vi "oa_Convert Waveform Reference Data Sample Rate (1 Channel).vi"(0 "resampled signal":cluster{"r0":dbl, "dr":dbl, "Y":dbl[]}={"r0"=0.0, "dr"=1.0, "Y"=[]} {"r0" format="%.2p"; "dr" format="%.2p"; "Y" format="%.2f"}, 5 "baseline in":cluster{"r0":dbl, "dr":dbl, "Y":dbl[]}={"r0"=0.0, "dr"=1.0, "Y"=[]} {"r0" format="%.2p"; "dr" format="%.2p"; "Y" format="%.2f"}, 11 "error out in":errorcluster) -> (4 "resampled signal dup":cluster{"r0":dbl, "dr":dbl, "Y":dbl[]}={"r0"=0.0, "dr"=1.0, "Y"=[]} {"r0" format="%.2p"; "dr" format="%.2p"; "Y" format="%.2f"}, 6 "baseline in out":cluster{"r0":dbl, "dr":dbl, "Y":dbl[]}={"r0"=0.0, "dr"=1.0, "Y"=[]} {"r0" format="%.2p"; "dr" format="%.2p"; "Y" format="%.2f"}, 15 "error out":errorcluster)   [LabVIEW 2017, in "SoundVib_RefDataProcess.lvlib"]
uses:
  <vilib>/addons/Sound and Vibration/Order Analysis/Referece Data Processing/SoundVib_RefDataProcess.lvlib
  <vilib>/measure/maresamp.llb/Resample Waveform (single shot).vi
  <vilib>/measure/NI_MAPro.lvlib
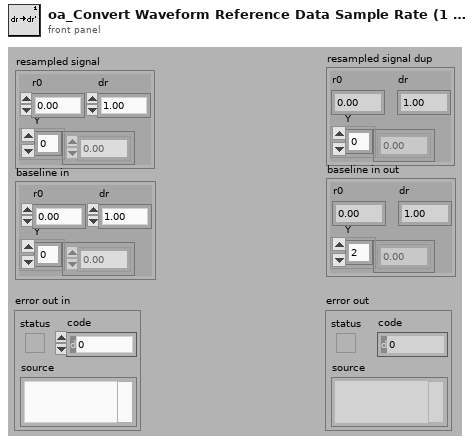
[diagram p1: front panel]
types:
  T1 = cluster{"alias rejection (dB)":dbl, "normalized bandwidth":dbl}
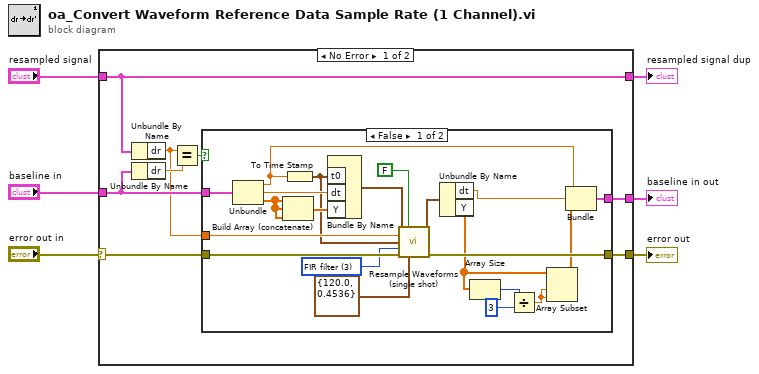
[diagram p0: block diagram]
diagram:
  n1 = case shown="No Error" "error out in" {
    selector: "error out in" -> [w12 w40]
    tunnel: [w11 w40] -> w5
    tunnel: "resampled signal" -> [w14 w39]
    tunnel: [w14 w39] -> w3
    tunnel: "baseline in" -> [w13 w38]
    tunnel: [w10 w38] -> w2
    frame No Error {
      n2 = Unbundle By Name(w14) -> ("dr"=w7:dbl)
      n3 = Unbundle By Name(w13) -> ("dr"=w9:dbl)
      n4 = Equal?(x=w7, y=w9) -> (x = y?=w8:bool)
      n5 = case shown="False" w8 {
        tunnel: w13 -> [w33 w37]
        tunnel: [w27 w37] -> w10
        tunnel: w12 -> [w35 w36]
        tunnel: [w34 w36] -> w11
        tunnel: w7 -> [w30 _]
        frame False {
          w26 = u16 3 items=["coerce", "linear", "spline", "FIR filter"] ("interpolation mode")
          n6 = Unbundle(w33) -> ("r0"=w23:dbl, "dr"=w32:dbl, "Y"=w17:dbl[])
          n7 = Build Array (concatenate)(w17, w17, w17) -> (w22:dbl[])
          n8 = To Time Stamp(1:w23) -> (0:w15:timestamp)
          n9 = Bundle By Name("t0"=w15, "dt"=w32, "Y"=w22) -> (w31:waveform(dbl))  [unwired: 1 in]
          n10 = call-poly <vilib>:"Resample Waveforms (single shot).vi"("waveform in"=w31, "open interval? (F)"=FALSE ("open interval? (T)"), "dt"=w30, "t0"=w15, "interpolation mode"=w26, "error in (no error)"=w35, "FIR filter specifications"=T1 {"alias rejection (dB)"=120.0, "normalized bandwidth"=0.4536}) -> ("resampled waveform out"=w29:waveform(dbl), "error out"=w34:errorcluster)  [unwired: 5 in, 2 out]
          n11 = Unbundle By Name(w29) -> ("dt"=w28:dbl, "Y"=w19:dbl[])
          n12 = Array Size(array=w19) -> (size(s)=w21:i32)
          n13 = Divide(x=w21, y=3) -> (x/y=w16:dbl)
          n14 = Array Subset(array=w19, index=w16, length=w16) -> (w18:dbl[])
          n15 = Bundle("r0"=w23, "dt"=w28, w18) -> (w27:cluster{"r0":dbl, "dt":dbl, dbl[]})  [unwired: 1 in]
        }
        frame True {
        }
      }
    }
    frame Error {
    }
  }
  "resampled signal dup" <- w3
  "baseline in out" <- w2
  "error out" <- w5
